vi "Gasteiler vor LIN Check Kalibrieren.vi"() -> ()   [LabVIEW 2020, in "Linearisierung v2.lvlib" / "Gasteiler.lvlib"]
uses:
  Gasteiler.lvlib
  AK-Komm Gasteiler/AK Komm Gasteiler.lvlib
  AK-Komm Gasteiler/Aktionen AK Komm.ctl
  Funktionstasten/Funktionstasten.lvlib
  Funktionstasten/Funktionstasten-Aktion.ctl
  AK-Komm Gasteiler/Alter Gasteiler/Alter Gasteiler.lvlib
  AK-Komm Gasteiler/Alter Gasteiler/Aktionen AK Komm_ALT.ctl
  Aktionen FGV Gasteiler Daten.ctl
  Allgemein/allgemeine Sub-VIs.lvlib
  Funktionstasten/Zustaende.ctl
  Visualisierungs Elemente/Button.ctl
  Visualisierungs Elemente/String - Ausgabefeld.ctl
panel:
  in  "Lin Check":T1
  out "Titelzeile":string
  out "Gasteiler Status":T2
  in  "Endpunkt":T1
  in  "Nullpunkt":T1
  in  "ABBRECHEN":T1
  # "Status Gasteiler"
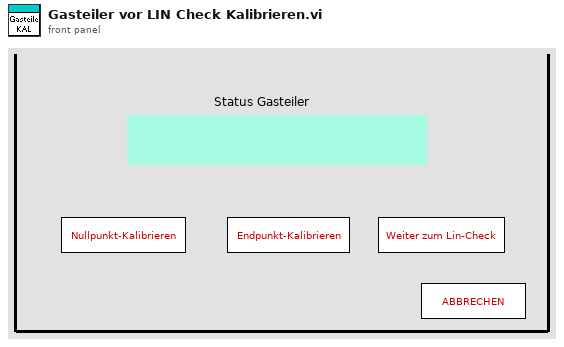
[diagram p1: front panel]
types:
  T1 = typedef "Button.ctl" = bool
  T2 = typedef "String - Ausgabefeld.ctl" = string
  T3 = typedef "Linearisierung v2.lvlib/Gasteiler.lvlib/Aktionen FGV Gasteiler Daten.ctl" = enum16{"lesen", "Gasteiler Daten", "Seriellen Param.", "MB-Endwert", "laden", "speichern", "Anforderung", "TCP", "Aufzeichnung Start"}
  T4 = typedef "Linearisierung v2.lvlib/Gasteiler.lvlib/AK Komm Gasteiler.lvlib/Aktionen AK Komm.ctl" = enum16{"lesen", "initialisieren", "beenden", "Status", "SMAN", "SREM", "STBY", "ASTF", "ASTZ", "SLST", "AGAT", "EGAK", "AGAK", "AKAK", "ADRU", "SKOP", "SVSA", "SVSZ", "SONO", "SAIR", "SNOX", "ANOX", "SSPL", "SRUC", "SLIN", "ALST"}
  T5 = typedef "Linearisierung v2.lvlib/Gasteiler.lvlib/AK Komm Gasteiler.lvlib/Alter Gasteiler.lvlib/Aktionen AK Komm_ALT.ctl" = enum16{"lesen", "initialisieren", "beenden", "SRES", "STBY", "SREM", "SMAN", "SLIN", "SLCH", "SLST", "SSPL", "AGAT", "ALST", "ASTZ", "ASTF", "AGAK", "EGAK"}
  T6 = typedef "Funktionstasten.lvlib/Zustaende.ctl" = enum16{"Standby", "Pause", "Eco", "Messen", "Kalibrieren", "Spülen Filter", "Spülen Leitung", "Umgebungsluft", "0-Gas", "Cal-Gas", "CG zu PNS", "-------------", "Init 1", "Init 2", "Init 3", "Init 4", "Messen vorbereiten", "Messen durchführen", "Exit"}
  T7 = typedef "Funktionstasten.lvlib/Funktionstasten-Aktion.ctl" = enum16{"Initialisieren", "Zustand setzen", "Taste gedrückt", "Fehler speichern", "Lesen", "Manuell", "Remote", "Bitparallel", "Samplepoint", "Zeit Prüfen", "reset Umschalten"}
  T8 = typedef "Linearisierung v2.lvlib/GasteilerType.ctl" = u16
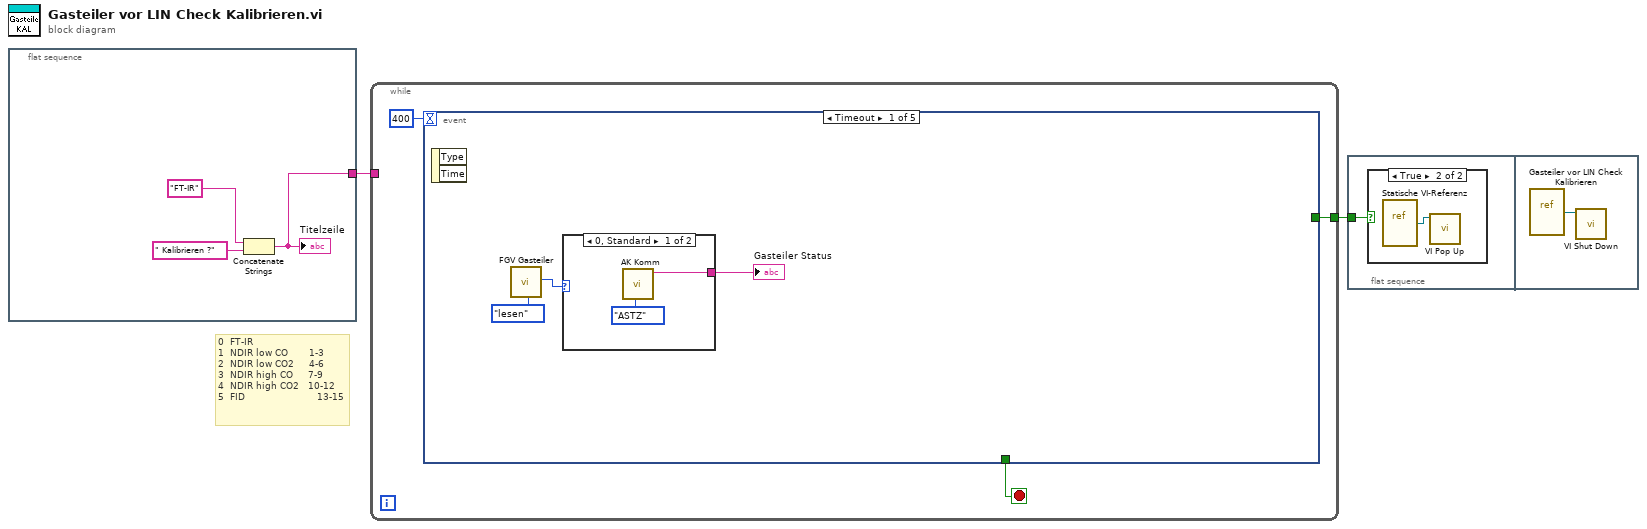
[diagram p0: block diagram]
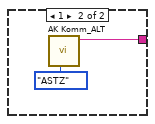
[diagram p3: hidden frame]
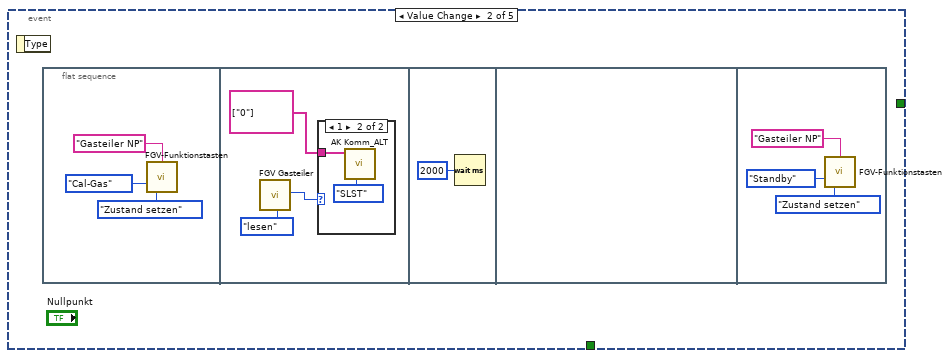
[diagram p4: hidden frame]
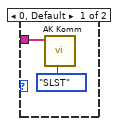
[diagram p5: hidden frame]
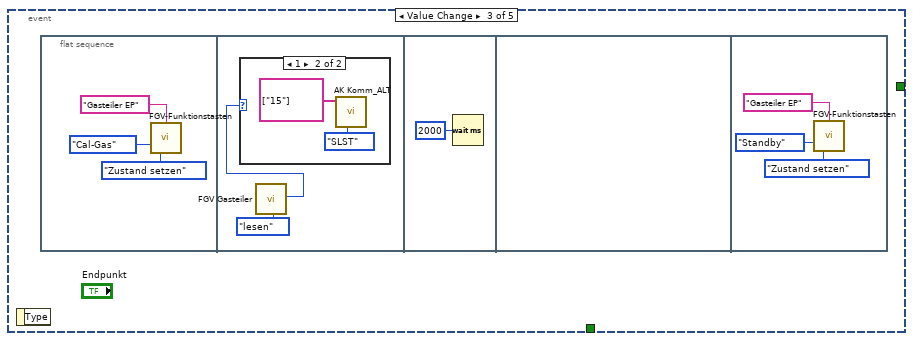
[diagram p6: hidden frame]
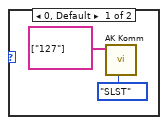
[diagram p7: hidden frame]
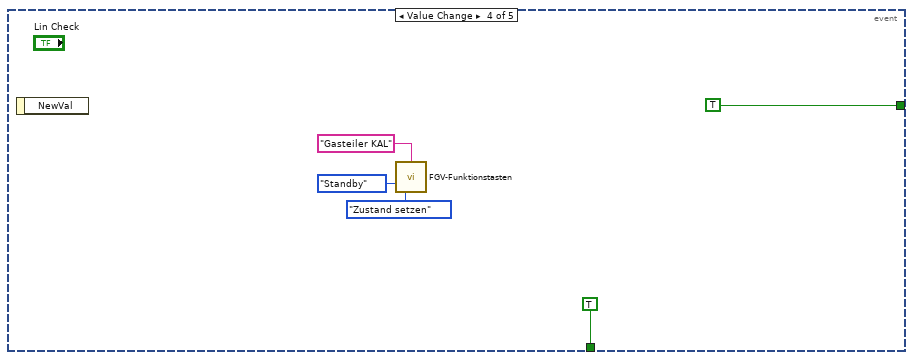
[diagram p8: hidden frame]
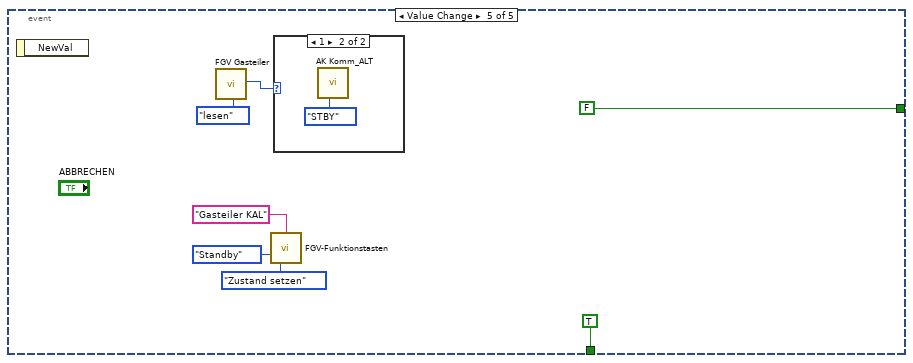
[diagram p9: hidden frame]
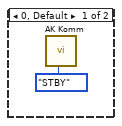
[diagram p10: hidden frame]
diagram:
  # "0  FT-IR\n1  NDIR low CO       1-3\n2  NDIR low CO2     4-6\n3  NDIR high CO     7-9\n4  NDIR high CO2   10-12\n5  FID                        13-15"
  n1 = flat-sequence {
    tunnel: [w3] -> w1
    frame #0 {
      n2 = Concatenate Strings("FT-IR" ("Titelzeile"), " Kalibrieren ?" ("String")) -> (w3:string)
      "Titelzeile" <- w3
    }
  }
  n3 = while {
    tunnel: [w6] -> w2
    tunnel: w1 -> [_]
    stop <- w7 stop-if-true
    n4 = event shown="[0] Timeout" {
      selector: _ -> [_ _ _ _ _]
      dyn-events: _ -> [_ _ _ _ _]
      timeout: 400 -> [_ _ _ _ _]
      tunnel: [_ _ _ TRUE ("ABBRECHEN") TRUE ("ABBRECHEN")] -> w7
      tunnel: [_ _ _ TRUE ("ABBRECHEN") FALSE ("ABBRECHEN")] -> w6
      event Timeout {
        n5 = event-data() -> ()  [unwired: 1 in, 2 out]
        n6 = call "FGV Gasteiler.vi"("Aktionen"=Aktionen_FGV_Gasteiler_Daten."lesen") -> ("Gasteiler Type"=w9:T8)  [unwired: 11 in, 7 out]
        n7 = case shown="0, Standard" w9 {
          tunnel: [w12 w14] -> w11
          frame 0, Default {
            n8 = call "AK Komm.vi"("Aktionen"=Aktionen_AK_Komm."ASTZ") -> ("Status"=w12:string)  [unwired: 5 in, 5 out]
          }
          frame 1 {
            n9 = call "AK Komm_ALT.vi"("Aktionen_ALT"=Aktionen_AK_Komm_ALT."ASTZ") -> ("Status"=w14:string)  [unwired: 6 in, 4 out]
          }
        }
        "Gasteiler Status" <- w11
      }
      event Value Change {
        n10 = event-data() -> ()  [unwired: 1 in, 1 out]
        n11 = flat-sequence {
          frame #0 {
            n12 = call "FGV-Funktionstasten.vi"("Herkunft"="Gasteiler NP", "Zustand"=Zustaende."Cal-Gas", "Aktion"=Funktionstasten-Aktion."Zustand setzen") -> ()  [unwired: 5 in, 8 out]
          }
          frame #1 {
            n13 = call "FGV Gasteiler.vi"("Aktionen"=Aktionen_FGV_Gasteiler_Daten."lesen") -> ("Gasteiler Type"=w19:T8)  [unwired: 11 in, 7 out]
            n14 = case shown="1" w19 {
              tunnel: string[] ["0"] ("Daten") -> [w22 w24]
              frame 0, Default {
                n15 = call "AK Komm.vi"("Aktionen"=Aktionen_AK_Komm."SLST", "Daten"=w22) -> ()  [unwired: 4 in, 6 out]
              }
              frame 1 {
                n16 = call "AK Komm_ALT.vi"("Aktionen_ALT"=Aktionen_AK_Komm_ALT."SLST", "Daten"=w24) -> ()  [unwired: 5 in, 5 out]
              }
            }
          }
          frame #2 {
            n17 = Wait (ms)(milliseconds to wait=u32 2000 ("Zu wartende ms")) -> ()  [unwired: 1 out]
          }
          frame #3 {
          }
          frame #4 {
            n18 = call "FGV-Funktionstasten.vi"("Herkunft"="Gasteiler NP", "Zustand"=Zustaende."Standby", "Aktion"=Funktionstasten-Aktion."Zustand setzen") -> ()  [unwired: 5 in, 8 out]
          }
        }
      }
      event Value Change {
        n19 = event-data() -> ()  [unwired: 1 in, 1 out]
        n20 = flat-sequence {
          frame #0 {
            n21 = call "FGV-Funktionstasten.vi"("Herkunft"="Gasteiler EP", "Zustand"=Zustaende."Cal-Gas", "Aktion"=Funktionstasten-Aktion."Zustand setzen") -> ()  [unwired: 5 in, 8 out]
          }
          frame #1 {
            n22 = call "FGV Gasteiler.vi"("Aktionen"=Aktionen_FGV_Gasteiler_Daten."lesen") -> ("Gasteiler Type"=w33:T8)  [unwired: 11 in, 7 out]
            n23 = case shown="1" w33 {
              frame 0, Default {
                n24 = call "AK Komm.vi"("Aktionen"=Aktionen_AK_Komm."SLST", "Daten"=string[] ["127"]) -> ()  [unwired: 4 in, 6 out]
              }
              frame 1 {
                n25 = call "AK Komm_ALT.vi"("Aktionen_ALT"=Aktionen_AK_Komm_ALT."SLST", "Daten"=string[] ["15"]) -> ()  [unwired: 5 in, 5 out]
              }
            }
          }
          frame #2 {
            n26 = Wait (ms)(milliseconds to wait=u32 2000 ("Zu wartende ms")) -> ()  [unwired: 1 out]
          }
          frame #3 {
          }
          frame #4 {
            n27 = call "FGV-Funktionstasten.vi"("Herkunft"="Gasteiler EP", "Zustand"=Zustaende."Standby", "Aktion"=Funktionstasten-Aktion."Zustand setzen") -> ()  [unwired: 5 in, 8 out]
          }
        }
      }
      event Value Change {
        n28 = event-data() -> ()  [unwired: 1 in, 1 out]
        n29 = call "FGV-Funktionstasten.vi"("Herkunft"="Gasteiler KAL", "Zustand"=Zustaende."Standby", "Aktion"=Funktionstasten-Aktion."Zustand setzen") -> ()  [unwired: 5 in, 8 out]
      }
      event Value Change {
        n30 = event-data() -> ()  [unwired: 1 in, 1 out]
        n31 = call "FGV Gasteiler.vi"("Aktionen"=Aktionen_FGV_Gasteiler_Daten."lesen") -> ("Gasteiler Type"=w49:T8)  [unwired: 11 in, 7 out]
        n32 = call "FGV-Funktionstasten.vi"("Herkunft"="Gasteiler KAL", "Zustand"=Zustaende."Standby", "Aktion"=Funktionstasten-Aktion."Zustand setzen") -> ()  [unwired: 5 in, 8 out]
        n33 = case shown="1" w49 {
          frame 0, Default {
            n34 = call "AK Komm.vi"("Aktionen"=Aktionen_AK_Komm."STBY") -> ()  [unwired: 5 in, 6 out]
          }
          frame 1 {
            n35 = call "AK Komm_ALT.vi"("Aktionen_ALT"=Aktionen_AK_Komm_ALT."STBY") -> ()  [unwired: 6 in, 5 out]
          }
        }
      }
    }
  }
  n36 = flat-sequence {
    tunnel: w2 -> [w57]
    frame #0 {
      n37 = case shown="True" w57 {
        frame False {
        }
        frame True {
          n38 = vi-ref "Statische VI-Referenz"() -> ("vi reference"=w58:refnum<vi>)
          n39 = call "VI Pop Up.vi"("VI Referenz"=w58) -> ()  [unwired: 11 in]
        }
      }
    }
    frame #1 {
      n40 = vi-ref "Gasteiler vor LIN Check Kalibrieren.vi"() -> (w59:refnum<vi>)
      n41 = call "VI Shut Down.vi"("VI Referenz"=w59) -> ()  [unwired: 11 in]
    }
  }
